vi "Global 2.vi"() -> ()   [LabVIEW 2017]
panel:
  out "Exit?":bool
  out "Exit":bool
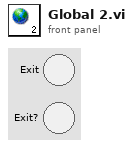
[diagram p1: front panel]
diagram:
